vi "Begin.vi"(8 "error in":errorcluster) -> (0 "error out":errorcluster)   [LabVIEW 2014]
doc: "Called before other user functions, this VI is expected to open initial I/O refnums, load in file data, and do all program initialization. Notice that the <B>error out</B> terminal is simply used for data flow. Wiring it to other structures or subVIs ensures that this VI runs first."
uses:
  <vilib>/Rock Robotics/WPI/DriverStation/WPI_DriverStationRobotMode2.ctl
  <vilib>/Rock Robotics/SystemInterfaces/DIO/FPGA_DIOPWMChannel.ctl
  <vilib>/Rock Robotics/WPI/SafetyOutput/WPI_SafetyOutputConfigMenu.ctl
  <vilib>/Rock Robotics/WPI/Joystick/WPI_JoystickDeviceEnum.ctl
  <vilib>/Rock Robotics/WPI/Solenoid/WPI_SolenoidChannel.ctl
  <vilib>/Rock Robotics/SystemInterfaces/DIO/FPGA_DIORelayChannel.ctl
  <vilib>/Rock Robotics/WPI/Relay/WPI_RelayDirection.ctl
  <vilib>/Rock Robotics/SystemInterfaces/DIO/FPGA_DIOChannel.ctl
  <vilib>/Rock Robotics/WPI/Encoder/WPI_EncoderType.ctl
  <vilib>/Rock Robotics/SystemInterfaces/AI/FPGA_AIChannel.ctl
  <vilib>/Rock Robotics/SystemInterfaces/AI/FPGA_AIGyroChannel.ctl
  Robot Global Data.vi
  <vilib>/Rock Robotics/Network Tables/SD Write String Array.vi
  <vilib>/Rock Robotics/WPI/RobotDrive/WPI_RobotDriveOpen2MotorWithTalon.vi
  <vilib>/Rock Robotics/WPI/MotorControl/WPI_MotorControlOpen Talon.vi
  <vilib>/Rock Robotics/WPI/Solenoid/WPI_SolenoidOpenDouble.vi
  <vilib>/Rock Robotics/WPI/Counter/WPI_CounterDigitalInputToDigitalSource.vi
  <vilib>/Rock Robotics/WPI/Ultrasonic/WPI_SonarMB1010AnalogOpen.vi
  <vilib>/Rock Robotics/WPI/Ultrasonic/WPI_SonarMB1010AnalogRefNum Registry Set.vi
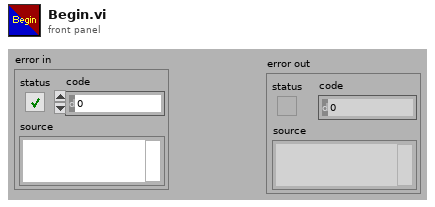
[diagram p1: front panel]
types:
  T1 = typedef "WPI_EncoderType.ctl" = enum16{"1x", "2x", "4x"}
  T2 = typedef "FPGA_AIGyroChannel.ctl" = enum8{"AI 0", "AI 1", "Invalid"}
  T3 = typedef "FPGA_AIChannel.ctl" = enum8{"AI 0", "AI 1", "AI 2", "AI 3", "AI MXP 0", "AI MXP 1", "AI MXP 2", "AI MXP 3", "Invalid"}
  T4 = typedef "FPGA_DIOChannel.ctl" = enum8{"DIO 0", "DIO 1", "DIO 2", "DIO 3", "DIO 4", "DIO 5", "DIO 6", "DIO 7", "DIO 8", "DIO 9", "DIO MXP 0", "DIO MXP 1", "DIO MXP 2", "DIO MXP 3", "DIO MXP 4", "DIO MXP 5", "DIO MXP 6", "DIO MXP 7", "DIO MXP 8", "DIO MXP 9", "DIO MXP 10", "DIO MXP 11", "DIO MXP 12", "DIO MXP 13", "DIO MXP 14", "DIO MXP 15", "Invalid"}
  T5 = typedef "WPI_RelayDirection.ctl" = enum16{"Both directions", "Forward only", "Reverse only"}
  T6 = typedef "FPGA_DIORelayChannel.ctl" = enum8{"Relay 0", "Relay 1", "Relay 2", "Relay 3", "Invalid"}
  T7 = typedef "WPI_SolenoidChannel.ctl" = enum8{"Solenoid 0", "Solenoid 1", "Solenoid 2", "Solenoid 3", "Solenoid 4", "Solenoid 5", "Solenoid 6", "Solenoid 7", "Invalid"}
  T8 = typedef "FPGA_DIOPWMChannel.ctl" = enum8{"PWM 0", "PWM 1", "PWM 2", "PWM 3", "PWM 4", "PWM 5", "PWM 6", "PWM 7", "PWM 8", "PWM 9", "PWM MXP 0", "PWM MXP 1", "PWM MXP 2", "PWM MXP 3", "PWM MXP 4", "PWM MXP 5", "PWM MXP 6", "PWM MXP 7", "PWM MXP 8", "PWM MXP 9", "Invalid"}
  T9 = typedef "WPI_JoystickDeviceEnum.ctl" = enum16{"USB 0", "USB 1", "USB 2", "USB 3", "USB 4", "USB 5"}
  T10 = typedef "WPI_SafetyOutputConfigMenu.ctl" = enum16{"Enable", "Disable"}
  T11 = typedef "WPI_DriverStationRobotMode2.ctl" = enum16{"Autonomous Disabled", "Autonomous Enabled", "Teleop Disabled", "Teleop Enabled", "Disconnected", "Finish", "Test Disabled", "Test Enabled", "Emergency Stopped"}
  T12 = typedef "WPI_MotorControlDeviceRef.ctl" = cluster{"DeviceStatus":errorcluster, "Type":T13, "PWM":cluster{"Controller":T14, "PWM Channel":T8, "DeadBand":T15}, "CAN":cluster{"Device Number":u8, "Control Mode":T16, "Semaphore":T17, "Max Vout":dbl, "TalonSRX Control Mode":T18}, "Invert":bool, "TransformRef":T19, "InvTransformRef":T19}
  T13 = typedef "WPI_MotorControlType.ctl" = enum16{"PWM", "CAN", "CANTalonSRX"}
  T14 = typedef "FPGA_TypedefDigitalModule.ctl" = enum16{"Controller 1"}
  T15 = typedef "WPI_PWMDeadband.ctl" = cluster{"Name":string, "maxPositivePwm":i32, "minPositivePwm":i32, "centerPwm":i32, "maxNegativePwm":i32, "minNegativePwm":i32, "angularRange":u16}
  T16 = typedef "WPI_CANJaguar_ControlMode.ctl" = enum8{"Percent VBus", "Current", "Speed", "Position", "Voltage"}
  T17 = typedef "Semaphore RefNum" = refnum<k1>
  T18 = typedef "WPI_CANTalonSRX_APIControlMode.ctl" = enum8{"Percent VBus", "Speed", "Position", "Slave", "Unchanged / Invalid"}
  T19 = typedef "WPI_PWMTransform_ConPane.ctl" = refnum<vi>
  T20 = typedef "WPI_RelayDevRef.ctl" = cluster{"DevStatus":errorcluster, "Relay Channel":T6, "Controller":T14, "Relay Direction":T5}
  T21 = typedef "WPI_DigitalInputDevRef.ctl" = cluster{"DevStatus":errorcluster, "DIO Channel":T4, "Controller":T14}
  T22 = typedef "WPI_RobotDriveDevRef.ctl" = cluster{"DevStatus":errorcluster, "Motors[]":T12[], "Square Inputs":bool, "Max Output":dbl}
  T23 = typedef "FPGA_CounterEncoderSourceConvertionLVSourceType.ctl" = cluster{"DevStatus":errorcluster, "AnalogTriggerMode?":bool, "DigitalMode":cluster{"Controller":T14, "DIO Channel":T24}, "AnalogTriggerMode":cluster{"AnalogTriggerIndex":T25, "OutputType":T26}}
  T24 = typedef "FPGA_DIODigitalSourceChannel.ctl" = enum8{"DIO 0", "DIO 1", "DIO 2", "DIO 3", "DIO 4", "DIO 5", "DIO 6", "DIO 7", "DIO 8", "DIO 9", "DIO MXP 0", "DIO MXP 1", "DIO MXP 2", "DIO MXP 3", "DIO MXP 4", "DIO MXP 5", "DIO MXP 6", "DIO MXP 7", "DIO MXP 8", "DIO MXP 9", "DIO MXP 10", "DIO MXP 11", "DIO MXP 12", "DIO MXP 13", "DIO MXP 14", "DIO MXP 15", "Disabled"}
  T25 = typedef "FPGA_AnalogTriggerIndex.ctl" = enum8{"Trig 0", "Trig 1", "Trig 2", "Trig 3", "Trig 4", "Trig 5", "Trig 6", "Trig 7", "Invalid"}
  T26 = typedef "FPGA_AnalogTriggerOutType.ctl" = enum16{"InWindow", "TriggerState", "Rising", "Falling"}
  T27 = typedef "WPI_EncoderDevRef.ctl" = cluster{"DevStatus":errorcluster, "EncoderIndex":T28, "CounterIndex":T29, "DistancePerCount":dbl, "Decoding Type":T1}
  T28 = typedef "FPGA_EncoderIdx.ctl" = enum8{"Enc 0", "Enc 1", "Enc 2", "Enc 3", "Enc 4", "Enc 5", "Enc 6", "Enc 7", "Invalid"}
  T29 = typedef "FPGA_CounterCtrSystemIndex.ctl" = enum8{"Ctr 0", "Ctr 1", "Ctr 2", "Ctr 3", "Ctr 4", "Ctr 5", "Ctr 6", "Ctr 7", "Invalid"}
  T30 = typedef "WPI_GyroDevRef.ctl" = cluster{"DevStatus":errorcluster, "Analog Module":T31, "Analog Channel":T3, "Offset":dbl, "Gain (VoltsPerDegree/Second)":dbl}
  T31 = typedef "FPGA_TypedefAnalogModule.ctl" = enum16{"Controller 1"}
  T32 = typedef "WPI_SonarMB1010AnalogDeviceRef.ctl" = cluster{"AIDeviceRef":T33, "Scaling factor (V/in)":dbl, "Average Bits":u8}
  T33 = typedef "WPI_AnalogChannelDevRef.ctl" = cluster{"DevStatus":errorcluster, "Controller":T31, "Analog Channel":T3}
  T34 = typedef "WPI_JoystickDevRef.ctl" = cluster{"Device":T9}
  T35 = typedef "WPI_SolenoidDevRef.ctl" = cluster{"DevStatus":errorcluster, "Pneumatics Control Module":u8, "Forward Solenoid Channel":T7, "Reverse Solenoid Channel":T7}
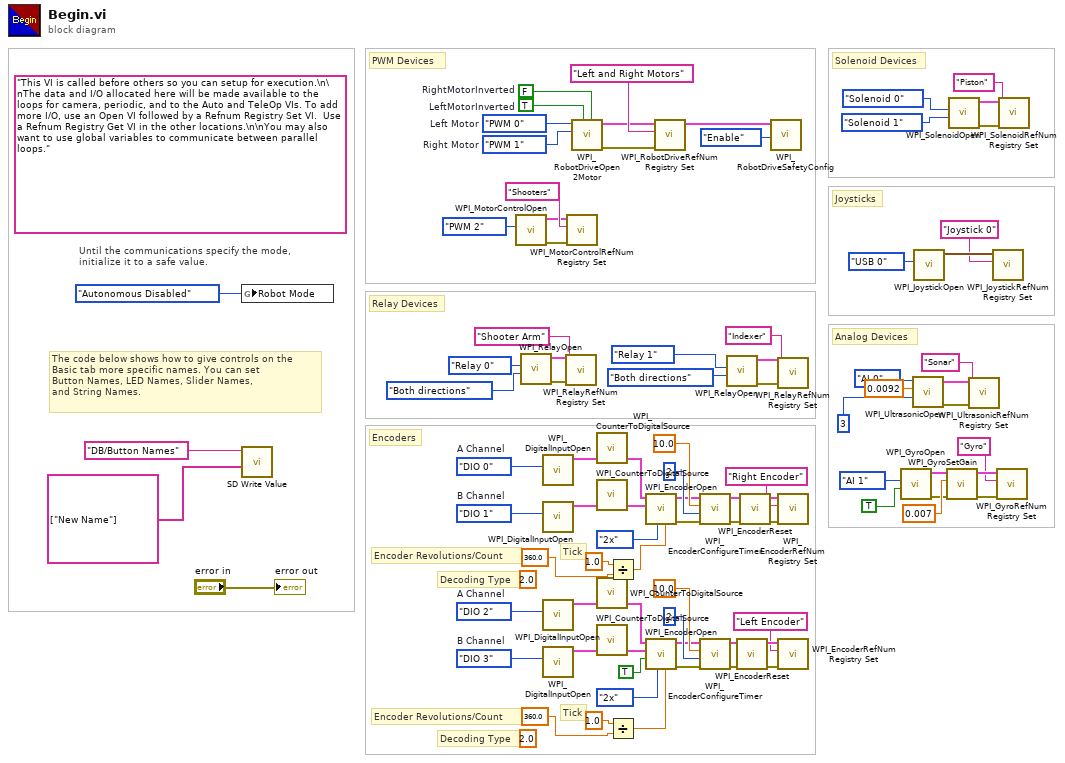
[diagram p0: block diagram]
diagram:
  (unwired) 2.0 ("Minimum Rate")
  (unwired) 2.0 ("Minimum Rate")
  w43 = FPGA_DIOChannel."DIO 3"  # B Channel
  w42 = FPGA_DIOChannel."DIO 2"  # A Channel
  w32 = FPGA_DIOChannel."DIO 1"  # B Channel
  w33 = FPGA_DIOChannel."DIO 0"  # A Channel
  w7 = FPGA_DIOPWMChannel."PWM 1"  # Right Motor
  w6 = FPGA_DIOPWMChannel."PWM 0"  # Left Motor
  w2 = TRUE  # LeftMotorInverted
  w1 = FALSE  # RightMotorInverted
  (unwired) "This VI is called before others so you can setup for execution.\n\nThe data and I/O allocated here will be made available to the loops for camera, periodic, and to the Auto and TeleOp VIs. To add more I/O, use an Open VI followed by a Refnum Registry Set VI.  Use a Refnum Registry Get VI in the other locations.\n\nYou may also want to use global variables to communicate between parallel loops."
  # "Tick"
  # "Decoding Type"
  # "Encoder Revolutions/Count"
  # "Tick"
  # "Decoding Type"
  # "Encoder Revolutions/Count"
  # "Analog Devices"
  # "Encoders"
  # "Joysticks"
  # "Solenoid Devices"
  # "Relay Devices"
  # "PWM Devices"
  # "The code below shows how to give controls on the\nBasic tab more specific names. You can set\nButton Names, LED Names, Slider Names,\nand String Names."
  # "Until the communications specify the mode,\ninitialize it to a safe value."
  n1 = global write "Robot Global Data.vi" "Robot Mode"(WPI_DriverStationRobotMode2."Autonomous Disabled" ("Robot Mode")) -> ()
  n2 = call-poly <vilib>:"SD Write Value.vi"("String Array"=string[] ["New Name"], "Name"="DB/Button Names") -> ()  [unwired: 8 in, 2 out]
  n3 = call-poly <vilib>:"WPI_MotorControlOpen.vi"("PWM Channel"=FPGA_DIOPWMChannel."PWM 2") -> ("error out"=w13:errorcluster, "MotorControlDeviceRef"=w14:T12)  [unwired: 9 in]
  n4 = call <vilib>:"WPI_RelayOpen.vi"("Relay Direction"=WPI_RelayDirection."Both directions", "Relay Channel"=FPGA_DIORelayChannel."Relay 0") -> ("error out"=w22:errorcluster, "RelayDevRef"=w23:T20)  [unwired: 8 in]
  n5 = call <vilib>:"WPI_DigitalInputOpen.vi"("DIO Channel"=w33) -> ("DigitalInputDevRef"=w36:T21)  [unwired: 2 in, 8 out]
  n6 = call <vilib>:"WPI_DigitalInputOpen.vi"("DIO Channel"=w32) -> ("DigitalInputDevRef"=w35:T21)  [unwired: 2 in, 8 out]
  n7 = call <vilib>:"WPI_DigitalInputOpen.vi"("DIO Channel"=w42) -> ("DigitalInputDevRef"=w39:T21)  [unwired: 2 in, 8 out]
  n8 = call <vilib>:"WPI_DigitalInputOpen.vi"("DIO Channel"=w43) -> ("DigitalInputDevRef"=w40:T21)  [unwired: 2 in, 8 out]
  n9 = call <vilib>:"WPI_RelayRefNum Registry Set.vi"("error in (no error)"=w22, "refnum name"="Shooter Arm", "RelayDevRef"=w23) -> ()  [unwired: 7 in, 2 out]
  n10 = call <vilib>:"WPI_MotorControlRefNum Registry Set.vi"("error in (no error)"=w13, "refnum name"="Shooters", "MotorControlDevRef"=w14) -> ()  [unwired: 7 in, 2 out]
  n11 = call-poly <vilib>:"WPI_RobotDriveOpen2Motor.vi"("Right Motor Inverted"=w1, "Left Motor Inverted"=w2, "Right Motor"=w7, "Left Motor"=w6) -> ("error out"=w5:errorcluster, "RobotDriveDevRef"=w3:T22)  [unwired: 1 in, 5 out]
  n12 = call-poly <vilib>:"WPI_CounterToDigitalSource.vi"("DigitalInputDevRef"=w36) -> ("Digital Source"=w37:T23)  [unwired: 6 out]
  n13 = call-poly <vilib>:"WPI_CounterToDigitalSource.vi"("DigitalInputDevRef"=w35) -> ("Digital Source"=w34:T23)  [unwired: 6 out]
  n14 = call-poly <vilib>:"WPI_CounterToDigitalSource.vi"("DigitalInputDevRef"=w39) -> ("Digital Source"=w38:T23)  [unwired: 6 out]
  n15 = call-poly <vilib>:"WPI_CounterToDigitalSource.vi"("DigitalInputDevRef"=w40) -> ("Digital Source"=w41:T23)  [unwired: 6 out]
  n16 = Divide(x=1.0 ("Minimum Rate"), y=360.0 ("Minimum Rate")) -> (x/y=w68:dbl)
  n17 = Divide(x=1.0 ("Minimum Rate"), y=360.0 ("Minimum Rate")) -> (x/y=w66:dbl)
  n18 = call <vilib>:"WPI_EncoderOpen.vi"("DistancePerCount"=w68, "Decoding Type"=WPI_EncoderType."2x", "BSource"=w34, "ASource"=w37) -> ("error out"=w45:errorcluster, "EncoderDevRef"=w46:T27)  [unwired: 4 in, 2 out]
  n19 = call <vilib>:"WPI_EncoderOpen.vi"("DistancePerCount"=w66, "Decoding Type"=WPI_EncoderType."2x", "Invert Direction (False)"=TRUE, "BSource"=w41, "ASource"=w38) -> ("error out"=w48:errorcluster, "EncoderDevRef"=w47:T27)  [unwired: 3 in, 2 out]
  n20 = call <vilib>:"WPI_RobotDriveRefNum Registry Set.vi"("error in (no error)"=w5, "refnum name"="Left and Right Motors", "RobotDriveDevRef"=w3) -> ("RobotDriveDevRef"=w8:T22)  [unwired: 8 out]
  n21 = call <vilib>:"WPI_EncoderConfigureTimer.vi"("error in (no error)"=w45, "Number Samples to Average"=u8 2, "Minimum Rate"=10.0, "EncoderDevRef"=w46) -> ("error out"=w77:errorcluster, "EncoderDevRef"=w76:T27)  [unwired: 6 in]
  n22 = call <vilib>:"WPI_EncoderConfigureTimer.vi"("error in (no error)"=w48, "Number Samples to Average"=u8 2, "Minimum Rate"=10.0, "EncoderDevRef"=w47) -> ("error out"=w74:errorcluster, "EncoderDevRef"=w75:T27)  [unwired: 6 in]
  n23 = call <vilib>:"WPI_RelayOpen.vi"("Relay Direction"=WPI_RelayDirection."Both directions", "Relay Channel"=FPGA_DIORelayChannel."Relay 1") -> ("error out"=w27:errorcluster, "RelayDevRef"=w28:T20)  [unwired: 8 in]
  n24 = call <vilib>:"WPI_EncoderReset.vi"("error in (no error)"=w74, "EncoderDevRef"=w75) -> ("error out"=w79:errorcluster, "EncoderDevRef"=w78:T27)  [unwired: 8 in]
  n25 = call <vilib>:"WPI_EncoderReset.vi"("error in (no error)"=w77, "EncoderDevRef"=w76) -> ("error out"=w72:errorcluster, "EncoderDevRef"=w73:T27)  [unwired: 8 in]
  n26 = call <vilib>:"WPI_RobotDriveSafetyConfig.vi"("mode"=WPI_SafetyOutputConfigMenu."Enable", "RobotDriveDevRef"=w8) -> ()  [unwired: 8 in, 2 out]
  n27 = call <vilib>:"WPI_RelayRefNum Registry Set.vi"("error in (no error)"=w27, "refnum name"="Indexer", "RelayDevRef"=w28) -> ()  [unwired: 7 in, 2 out]
  n28 = call <vilib>:"WPI_EncoderRefNum Registry Set.vi"("error in (no error)"=w72, "refnum name"="Right Encoder", "EncoderDevRef"=w73) -> ()  [unwired: 7 in, 2 out]
  n29 = call <vilib>:"WPI_EncoderRefNum Registry Set.vi"("error in (no error)"=w79, "refnum name"="Left Encoder", "EncoderDevRef"=w78) -> ()  [unwired: 7 in, 2 out]
  n30 = call <vilib>:"WPI_GyroOpen.vi"("Calibrate On Open"=TRUE, "Analog Channel"=FPGA_AIGyroChannel."AI 1") -> ("error out"=w60:errorcluster, "GyroDevRef"=w59:T30)  [unwired: 7 in, 1 out]
  n31 = call-poly <vilib>:"WPI_UltrasonicOpen.vi"("Average Bits"=u8 3, "Scaling factor (V/in)"=0.0092, "Analog Channel"=FPGA_AIChannel."AI 0") -> ("error out"=w53:errorcluster, "SonarMB1010AnalogDevRef"=w54:T32)  [unwired: 7 in]
  n32 = call <vilib>:"WPI_JoystickOpen.vi"("JoystickDevice"=WPI_JoystickDeviceEnum."USB 0") -> ("JoystickDevRef"=w11:T34)  [unwired: 10 in]
  n33 = call <vilib>:"WPI_GyroSetGain.vi"("error in (no error)"=w60, "Gain (VoltsPerDegree/Second)"=0.007, "GyroDevRef"=w59) -> ("error out"=w61:errorcluster, "GyroDevRef"=w62:T30)  [unwired: 7 in]
  n34 = call-poly <vilib>:"WPI_SolenoidOpen.vi"("Reverse Solenoid Channel"=WPI_SolenoidChannel."Solenoid 1" ("Forward Solenoid Channel"), "Forward Solenoid Channel"=WPI_SolenoidChannel."Solenoid 0") -> ("error out"=w17:errorcluster, "SolenoidDevRef"=w18:T35)  [unwired: 8 in]
  n35 = call-poly <vilib>:"WPI_UltrasonicRefNum Registry Set.vi"("error in (no error)"=w53, "refnum name"="Sonar", "SonarMB1010AnalogDevRef"=w54) -> ()  [unwired: 7 in, 2 out]
  n36 = call <vilib>:"WPI_JoystickRefNum Registry Set.vi"("refnum name"="Joystick 0", "JoystickDevRef"=w11) -> ()  [unwired: 8 in, 2 out]
  n37 = call <vilib>:"WPI_GyroRefNum Registry Set.vi"("error in (no error)"=w61, "refnum name"="Gyro", "GyroDevRef"=w62) -> ()  [unwired: 7 in, 2 out]
  n38 = call <vilib>:"WPI_SolenoidRefNum Registry Set.vi"("error in (no error)"=w17, "refnum name"="Piston", "SolenoidDevRef"=w18) -> ()  [unwired: 7 in, 2 out]
  "error out" <- "error in"
